vi "程序运行时，改变控件标题.vi"() -> ()   [LabVIEW 2022 SP3]
doc: "本VI是为《我和LabVIEW》一书编写的示例。\n关于本书的介绍请参考网页：\nhttp://ruanqizhen.spaces.live.com/blog/cns!5852D4F797C53FB6!4310.entry"
panel:
  in  "停止":bool
  in  "输入值的含义":enum32{"长度", "重量"}(radio)
  out "变体":variant
  in  "数值":dbl caption="重量输入"
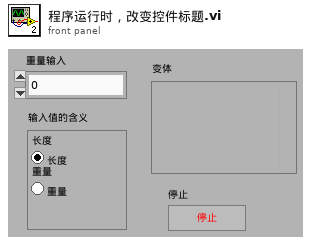
[diagram p1: front panel]
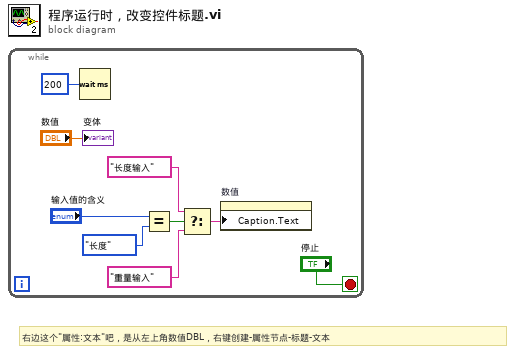
[diagram p0: block diagram]
diagram:
  # "右边这个\"属性:文本\"吧，是从左上角数值DBL，右键创建-属性节点-标题-文本"
  n1 = while {
    stop <- "停止" stop-if-true
    n2 = Wait (ms)(milliseconds to wait=u32 200 ("等待时间（毫秒）")) -> ()  [unwired: 1 out]
    n3 = Equal?(x="输入值的含义", y=enum32{"长度", "重量"}."长度") -> (x = y?=w4:bool)
    n4 = Select(t="长度输入", s=w4, f="重量输入") -> (s? t:f=w1:string)
    n5 = property on="数值" class="DigNum (严格)"("Caption.Text"=w1) -> ()  [unwired: 2 in, 2 out]
    "变体" <- "数值"
  }
